vi "SP Convert TPs to SPs.vi"(10 "T-Parameters":T2) -> (2 "SP Array":T1)   [LabVIEW 2011]
uses:
  TypeDefs/SP TP Data.ctl
  TypeDefs/SP Data.ctl
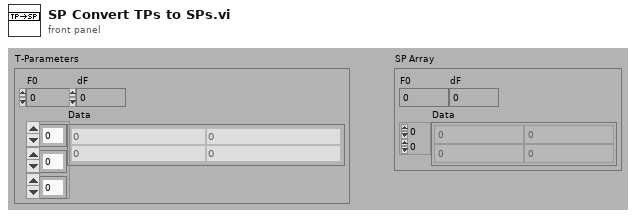
[diagram p1: front panel]
types:
  T1 = typedef "SP Data.ctl" = cluster{"F0":dbl, "dF":dbl, "Data":cdb[][]}
  T2 = typedef "SP TP Data.ctl" = cluster{"F0":dbl, "dF":dbl, "Data":cdb[][][]}
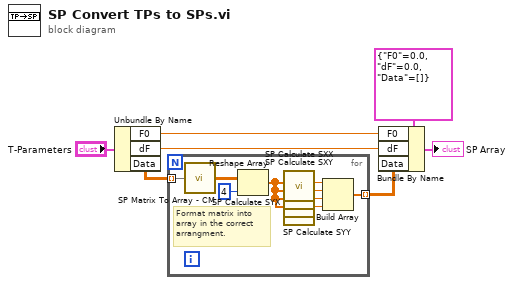
[diagram p0: block diagram]
diagram:
  n1 = Unbundle By Name("T-Parameters") -> ("F0"=w4:dbl, "dF"=w3:dbl, "Data"=w2:cdb[][][])
  n2 = for {
    tunnel: w2 -> [w11] mode=indexing
    tunnel: [w8] -> w1 mode=indexing
    # "Format matrix into\narray in the correct\narrangment."
    n3 = call "SP Matrix To Array - CM.vi"("Complex Matrix"=w11) -> ("Complex 2D Array"=w10:cdb[][])
    n4 = Reshape Array(w10, 4 ("dimension size")) -> (w9:cdb[])
    n5 = call "SP Calculate SXX.vi"("TP Array (TXX, TXY, TYX, TYY)"=w9) -> ("SXX"=w15:cdb)  [unwired: 10 out]
    n6 = call "SP Calculate SXY.vi"("TP Array (TXX, TXY, TYX, TYY)"=w9) -> ("SXY"=w14:cdb)  [unwired: 10 out]
    n7 = call "SP Calculate SYX.vi"("TP Array (TXX, TXY, TYX, TYY)"=w9) -> ("SYX"=w13:cdb)  [unwired: 10 out]
    n8 = call "SP Calculate SYY.vi"("TP Array (TXX, TXY, TYX, TYY)"=w9) -> ("SYY"=w12:cdb)  [unwired: 10 out]
    n9 = Build Array(w15, w14, w13, w12) -> (w8:cdb[])
  }
  n10 = Bundle By Name(cluster=T1 {"F0"=0.0, "dF"=0.0, "Data"=[]} ("SP Array"), "F0"=w4, "dF"=w3, "Data"=w1) -> (→"SP Array":T1)
